vi "S4P Data Processing old.vi"(0 "s4p path":path) -> (14 "frequency(Hz)":dbl[](array[numeric]), 16 "Sxx_R":dbl[][](array[numeric]), 18 "Sxx_I":dbl[][](array[numeric]), 19 "TXT_Data":string)   [LabVIEW 2011]
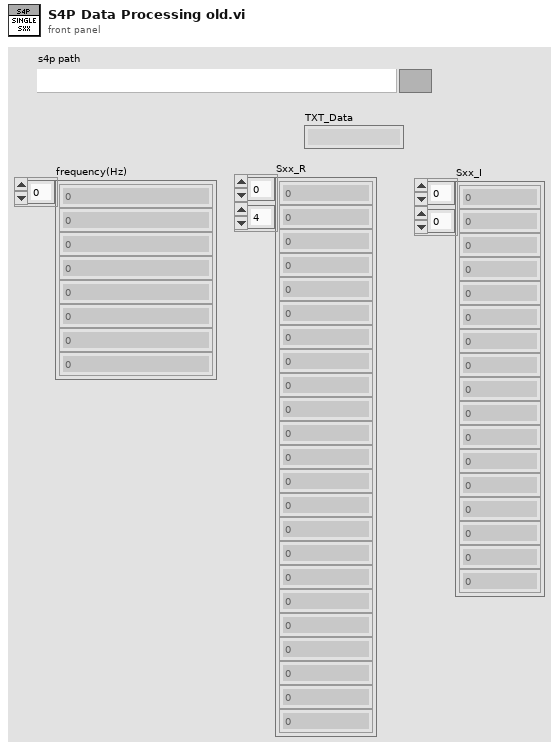
[diagram p1: front panel]
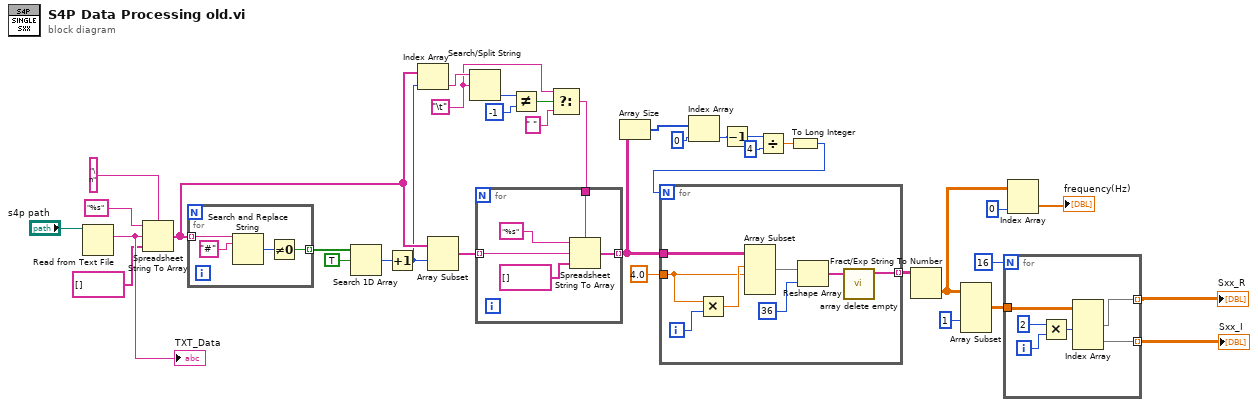
[diagram p0: block diagram]
diagram:
  w5 = "\t"
  n1 = Read from Text File(file (use dialog)="s4p path") -> (text=w36:string)  [unwired: 3 in, 3 out]
  "TXT_Data" <- w36
  n2 = Spreadsheet String To Array(delimiter (Tab)="\n" ("分隔符(Tab)"), format string="%s" ("格式字符串"), spreadsheet string=w36, array type (2D Dbl)=string[] []) -> (array=w11:string[])
  n3 = for {
    tunnel: w11 -> [w40] mode=indexing
    tunnel: [w37] -> w32 mode=indexing
    n4 = Search and Replace String(input string=w40, search string="#" ("搜索字符串")) -> (number of replacements=w38:i32)  [unwired: 6 in, 3 out]
    n5 = Not Equal To 0?(x=w38) -> (x != 0?=w37:bool)
  }
  n6 = Search 1D Array(1D array=w32, element=TRUE ("元素")) -> (index of element=w29:i32)  [unwired: 1 in]
  n7 = Increment(x=w29) -> (x+1=w10:i32)
  n8 = Index Array(array=w11, index=w10) -> (element=w9:string)
  n9 = Array Subset(array=w11, index=w10) -> (w28:string[])  [unwired: 1 in]
  n10 = Search/Split String(string=w9, search string/char (-)=w5) -> (offset of match=w8:i32)  [unwired: 1 in, 2 out]
  n11 = Not Equal?(x=w8, y=-1) -> (x != y?=w6:bool)
  n12 = Select(t=w5, s=w6, f=" " ("分隔符(Tab)")) -> (s? t:f=w3:string)
  n13 = for {
    tunnel: w28 -> [w45] mode=indexing
    tunnel: [w42] -> w19 mode=indexing
    tunnel: w3 -> [w41]
    n14 = Spreadsheet String To Array(delimiter (Tab)=w41, format string="%s" ("格式字符串"), spreadsheet string=w45, array type (2D Dbl)=string[] []) -> (array=w42:string[])
  }
  n15 = Array Size(array=w19) -> (size(s)=w18:i32[])
  n16 = Index Array(array=w18, index=0 ("索引")) -> (element=w16:i32)
  n17 = Decrement(x=w16) -> (x-1=w15:i32)
  n18 = Divide(x=w15, y=4) -> (x/y=w13:dbl)
  n19 = To Long Integer(number=w13) -> (32bit integer=w12:i32)
  n20 = for {
    N: w12 -> [_]
    tunnel: w19 -> [w53]
    tunnel: 4.0 ("y") -> [w48]
    tunnel: [w46] -> w25 mode=indexing
    i -> [w52]
    n21 = Multiply(x=w48, y=w52) -> (x*y=w51:dbl)
    n22 = Array Subset(array=w53, index (row)=w51, length (row)=w48) -> (w50:string[][])  [unwired: 2 in]
    n23 = Reshape Array(w50, 36 ("维数大小")) -> (w47:string[])
    n24 = call "array delete empty.vi"("input"=w47) -> ("output"=w46:string[])  [unwired: 10 in]
  }
  n25 = Fract/Exp String To Number(string=w25) -> (number=w24:dbl[][])  [unwired: 3 in, 1 out]
  n26 = Array Subset(array=w24, index (col)=1 ("索引")) -> (w22:dbl[][])  [unwired: 3 in]
  n27 = for {
    N: 16 -> [_]
    tunnel: w22 -> [w59]
    tunnel: [w55] -> w2 mode=indexing
    tunnel: [w54] -> w1 mode=indexing
    i -> [w58]
    n28 = Multiply(x=2, y=w58) -> (x*y=w56:i32)
    n29 = Index Array(array=w59, index (col) #1=w56) -> (element #1=w55:dbl[], element #2=w54:dbl[])  [unwired: 3 in]
  }
  "Sxx_R" <- w2
  "Sxx_I" <- w1
  n30 = Index Array(array=w24, index (col)=0 ("禁用的索引 (列)")) -> (element=→"frequency(Hz)":dbl[])  [unwired: 1 in]
